vi "Start REPL.vi"() -> ()   [LabVIEW 2016]
panel:
  in  "Control Name":string="Robot REPL"
  in  "Code Ref":refnum<vi>
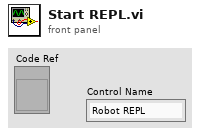
[diagram p1: front panel]
types:
  T1 = cluster{"VISA Refnum in":refnum<visa-resource-name>, "Python Code":string}[]
  T2 = cluster{"VISA Refnum in":refnum<visa-resource-name>, "Python Code":string}
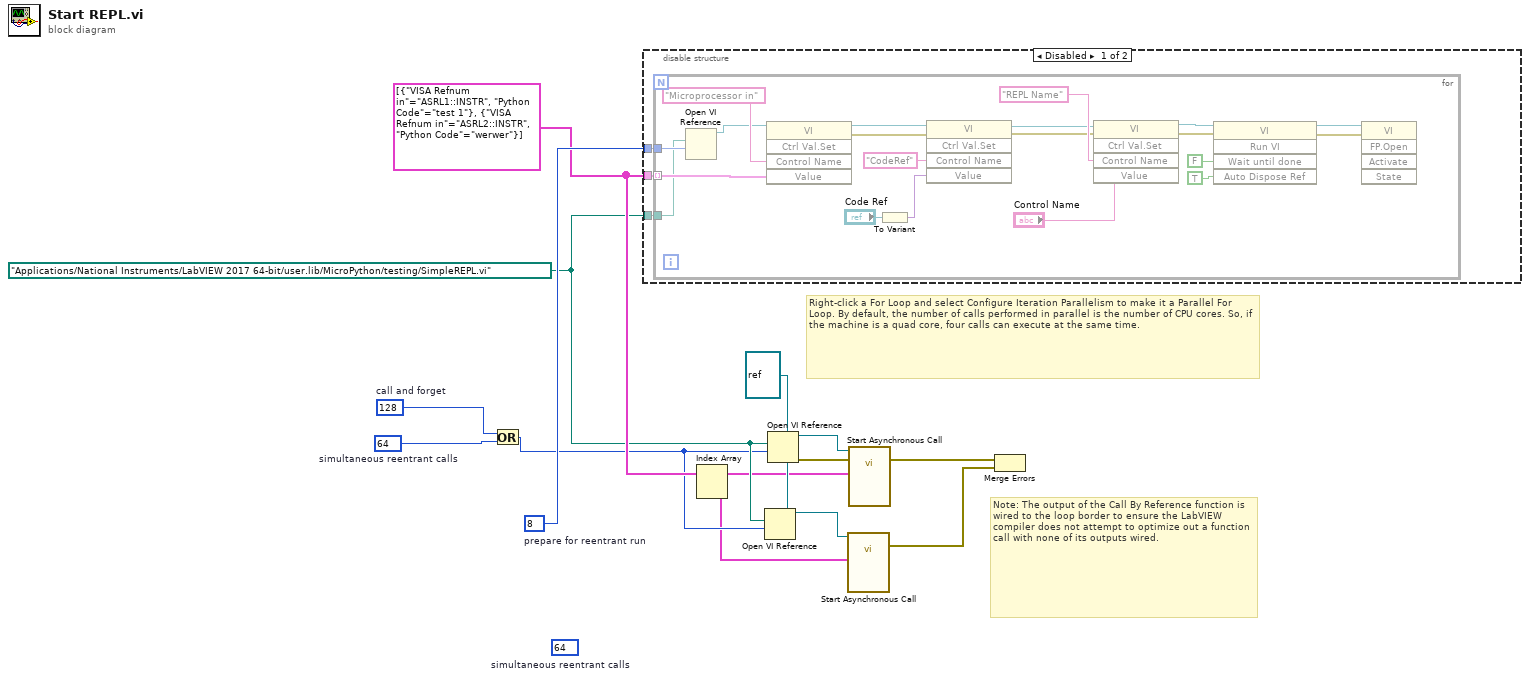
[diagram p0: block diagram]
diagram:
  (unwired) 64  # simultaneous reentrant calls
  w9 = T1 [{"VISA Refnum in"="ASRL1::INSTR", "Python Code"="test 1"}, {"VISA Refnum in"="ASRL2::INSTR", "Python Code"="werwer"}]
  w12 = 8  # prepare for reentrant run
  w13 = 64  # simultaneous reentrant calls
  w14 = 128  # call and forget
  w7 = path "/Applications/National Instruments/LabVIEW 2017 64-bit/user.lib/MicroPython/testing/SimpleREPL.vi" ("vi path")
  w6 = refnum<vi> refnum ("reference")
  # "Note: The output of the Call By Reference function is wired to the loop border to ensure the LabVIEW compiler does not attempt to optimize out a function call with none of its outputs wired."
  # "Right-click a For Loop and select Configure Iteration Parallelism to make it a Parallel For Loop. By default, the number of calls performed in parallel is the number of CPU cores. So, if the machine is a quad core, four calls can execute at the same time."
  n1 = Or(x=w14, y=w13) -> (x .or. y?=w5:i32)
  n2 = disable-structure shown="Disabled" {
    disable-tunnel: w12 -> [w17 _]
    disable-tunnel: w7 -> [w16 _]
    disable-tunnel: w9 -> [w15 _]
    frame Disabled {
      n3 = for {
        tunnel: w15 -> [w21] mode=indexing
        tunnel: w17 -> [w20]
        tunnel: w16 -> [w19]
        n4 = Open VI Reference(vi path=w19, options=w20) -> (vi reference=w18:refnum<vi>)  [unwired: 4 in, 1 out]
        n5 = invoke class="VI" method="Ctrl Val.Set"(reference=w18, "Control Name"="Microprocessor in", "Value"=w21) -> (reference out=w32:refnum<vi>, error out=w31:errorcluster)  [unwired: 2 in, 3 out]
        n6 = To Variant(anything="Code Ref") -> (Variant=w28:variant)
        n7 = invoke class="VI" method="Ctrl Val.Set"(reference=w32, error in=w31, "Control Name"="CodeRef", "Value"=w28) -> (reference out=w26:refnum<vi>, error out=w24:errorcluster)  [unwired: 1 in, 3 out]
        n8 = invoke class="VI" method="Ctrl Val.Set"(reference=w26, error in=w24, "Control Name"="REPL Name", "Value"="Control Name") -> (reference out=w25:refnum<vi>, error out=w23:errorcluster)  [unwired: 1 in, 3 out]
        n9 = invoke class="VI" method="Run VI"(reference=w25, error in=w23, "Wait until done"=FALSE ("Wait Until Done"), "Auto Dispose Ref"=TRUE ("Auto Dispose Reference")) -> (reference out=w36:refnum<vi>, error out=w37:errorcluster)  [unwired: 1 in, 3 out]
        n10 = invoke class="VI" method="FP.Open"(reference=w36, error in=w37) -> ()  [unwired: 3 in, 5 out]
      }
    }
    frame Enabled {
    }
  }
  n11 = Index Array(array=w9) -> (element #1=w2:T2, element #2=w1:T2)  [unwired: 2 in]
  n12 = Open VI Reference(type specifier VI Refnum (for type only)=w6, vi path=w7, options=w5) -> (vi reference=w4:refnum<vi>)  [unwired: 3 in, 1 out]
  n13 = Open VI Reference(type specifier VI Refnum (for type only)=w6, vi path=w7, options=w5) -> (vi reference=w3:refnum<vi>, error out=w11:errorcluster)  [unwired: 3 in]
  n14 = call-by-ref "Start Asynchronous Call"(reference=w4, "Microprocessor in"=w1) -> (error out=w8:errorcluster)  [unwired: 12 in, 1 out]
  n15 = call-by-ref "Start Asynchronous Call"(reference=w3, error in=w11, "Microprocessor in"=w2) -> (error out=w10:errorcluster)  [unwired: 11 in, 1 out]
  n16 = Merge Errors(w10, w8) -> ()  [unwired: 1 out]
